vi "HiPOT.vi"(8 "error in":errorcluster, 9 "Setting":T1={"dc voltage"=100, "high limit"=4e-07, "test time(s)"=3.0, "Channel"=""}, 10 "HiPOT Ref":string, 11 "Analog In":refnum<class "Analog In.lvclass">) -> (0 "error out":errorcluster, 2 "Measurements":dbl[](array[numeric]), 3 "Analog In out":refnum<class "Analog In.lvclass">)   [LabVIEW 2019, in "Code Modules.lvlib"]
uses:
  Code Modules.lvlib
  PPLs/Hardware Abstraction.lvlibp/Harware Abstraction/Analog In/Analog In.lvclass
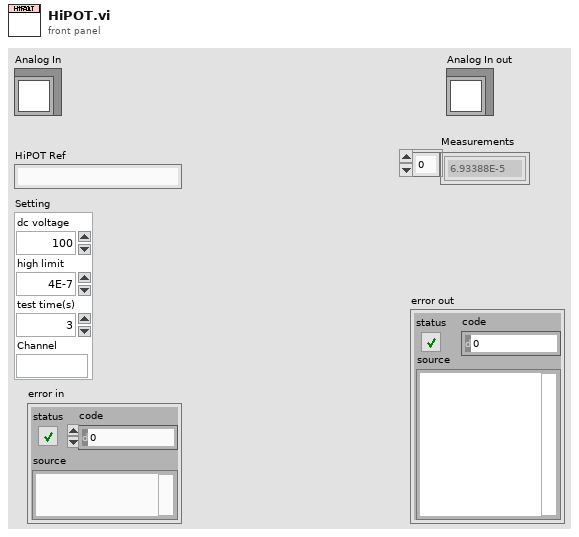
[diagram p1: front panel]
types:
  T1 = cluster{"dc voltage":i32, "high limit":dbl, "test time(s)":dbl, "Channel":string}
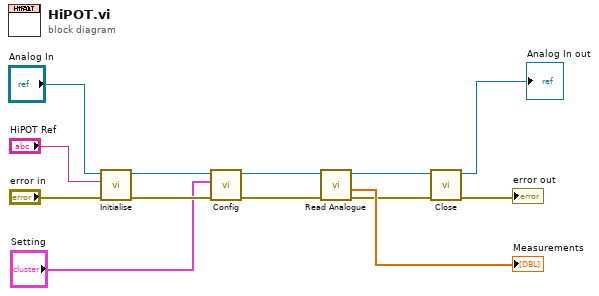
[diagram p0: block diagram]
diagram:
  n1 = call-dynamic "Initialise.vi"("error in (no error)"="error in", "Instrument Ref"="HiPOT Ref", "Instrument in"="Analog In") -> ("error out"=w10:errorcluster, "Instrument out"=w9:refnum<class "Analog In.lvclass">)  [unwired: 7 in]
  n2 = call-dynamic "Config.vi"("error in (no error)"=w10, "Setting"="Setting", "Analog In in"=w9) -> ("error out"=w7:errorcluster, "Analog In out"=w8:refnum<class "Analog In.lvclass">)  [unwired: 7 in]
  n3 = call-dynamic "Read Analogue.vi"("error in (no error)"=w7, "PS in"=w8) -> ("error out"=w4:errorcluster, "Measurements"=→"Measurements":dbl[], "PS out"=w5:refnum<class "Analog In.lvclass">)  [unwired: 6 in, 1 out]
  n4 = call-dynamic "Close.vi"("error in (no error)"=w4, "Instrument in"=w5) -> ("error out"=→"error out":errorcluster, "Instrument out"=→"Analog In out":refnum<class "Analog In.lvclass">)  [unwired: 8 in]
